vi "Set and Get Active Row Font.vi"(6 "Active Row":i32, 7 "Mode":T2, 8 "错误输入":errorcluster, 10 "Cell Font In":T1 caption="活动行:单元格字体", 11 "Listbox Ref":refnum<vi>) -> (0 "错误输出":errorcluster, 2 "Cell Font Out":T1 caption="活动行:单元格字体", 3 "Dup Listbox Ref":refnum<vi>)   [LabVIEW 2011, in "Listbox Tool.lvlib"]
uses:
  Listbox Tool.lvlib
  Custom Type/Read and Write Mode.ctl
  <vilib>/Utility/miscctls.llb/LVFontTypeDef.ctl
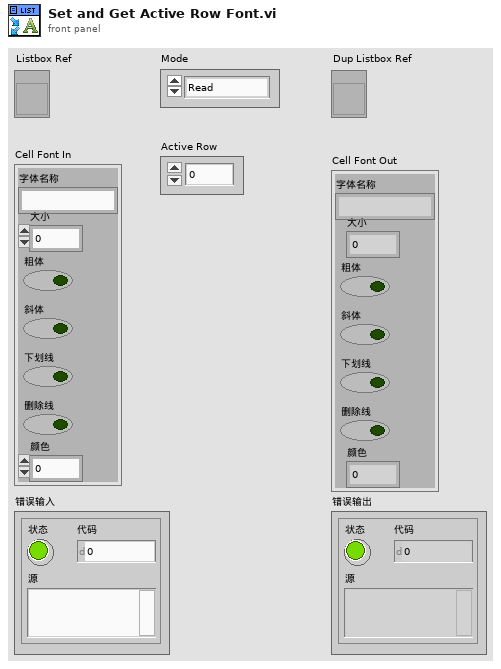
[diagram p1: front panel]
types:
  T1 = typedef "LVFontTypeDef.ctl" = cluster{"Font Name":string, "Size":u16, "Bold":bool, "Italic":bool, "Underline":bool, "Strikeout":bool, "Color":u32}
  T2 = typedef "Listbox Tool.lvlib/Read and Write Mode.ctl" = enum16{"Read", "Write"}
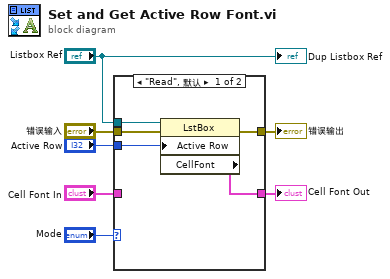
[diagram p0: block diagram]
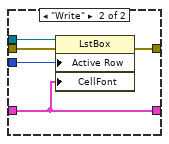
[diagram p2: hidden frame]
diagram:
  n1 = case shown="\"Read\", 默认" "Mode" {
    tunnel: "Active Row" -> [w12 w17]
    tunnel: "错误输入" -> [w11 w13]
    tunnel: [w10 w14] -> w4
    tunnel: "Listbox Ref" -> [w9 w16]
    tunnel: "Cell Font In" -> [_ w15]
    tunnel: [w8 w15] -> w1
    frame "Read", Default {
      n2 = property class="LstBox"(reference=w9, error in=w11, "Active Row"=w12) -> (error out=w10:errorcluster, "CellFont"=w8:T1)  [unwired: 1 out]
    }
    frame "Write" {
      n3 = property class="LstBox"(reference=w16, error in=w13, "Active Row"=w17, "CellFont"=w15) -> (error out=w14:errorcluster)  [unwired: 1 out]
    }
  }
  "错误输出" <- w4
  "Cell Font Out" <- w1
  "Dup Listbox Ref" <- "Listbox Ref"
